vi "srednia(SubVI).vi"(11 "input":dbl[](array[numeric])) -> (1 "RMS":dbl, 2 "kw":dbl, 3 "arytm":dbl)   [LabVIEW 2025]
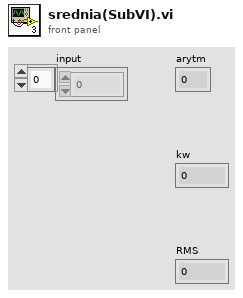
[diagram p1: front panel]
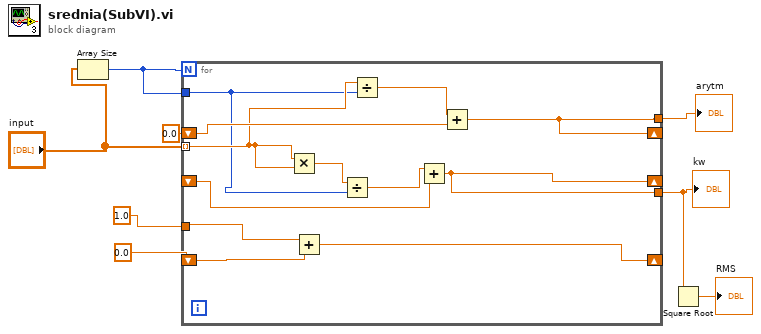
[diagram p0: block diagram]
diagram:
  n1 = Array Size(array="input") -> (size(s)=w5:i32)
  n2 = for {
    N: w5 -> [_]
    shift-right: [w19] -> _
    shift-left: 0.0 -> [w20]
    tunnel: [w16] -> w2
    tunnel: 1.0 ("x") -> [w18]
    tunnel: "input" -> [w14] mode=indexing
    tunnel: w5 -> [w12]
    shift-right: [w16] -> _
    shift-left: 0.0 -> [w15]
    shift-right: [w9] -> _
    shift-left: _ -> [w10]
    tunnel: [w9] -> w7
    n3 = Multiply(x=w14, y=w14) -> (x*y=w13:dbl)
    n4 = Add(x=w18, y=w20) -> (x+y=w19:dbl)
    n5 = Divide(x=w13, y=w12) -> (x/y=w11:dbl)
    n6 = Divide(x=w14, y=w12) -> (x/y=w17:dbl)
    n7 = Add(x=w11, y=w10) -> (x+y=w9:dbl)
    n8 = Add(x=w17, y=w15) -> (x+y=w16:dbl)
  }
  "arytm" <- w2
  "kw" <- w7
  n9 = Square Root(x=w7) -> (sqrt(x)=→"RMS":dbl)
